vi "InitFromCfgFile.vi"(8 "error in (no error)":errorcluster, 10 "configuration file path":path) -> (0 "error out":errorcluster, 3 "ByteQXAPIBase out":refnum<class "ByteQXAPIBase.lvclass">)   [LabVIEW 2019, in "ByteQXWebAPI.lvlib" / "ByteQXAPIBase.lvclass"]
doc: "Initialize the api connection based on the path of an ini file containing the configuration\n[Server]\nAPI Root = \"\"\nVersion = \"\"\nPort = 0\nBase URL = \"\"\nVerify server =\nAuth type = \nTimeout = 10000\n\n[Token]\nAuth = \"\""
uses:
  ByteQXAPIBase.lvclass
  <vilib>/Utility/config.llb/Read Key (U32).vi
  <vilib>/Utility/config.llb/Read Key (String).vi
  <vilib>/Utility/config.llb/NI_LVConfig.lvlib
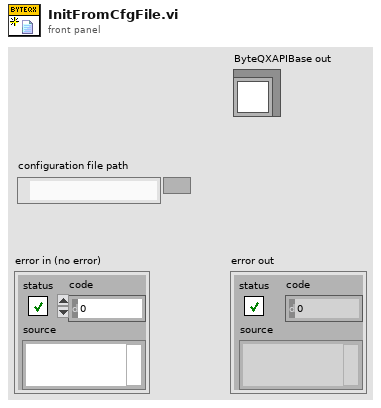
[diagram p1: front panel]
types:
  T1 = typedef "NI_LVConfig.lvlib/Config Data RefNum.ctl" = refnum<k1>
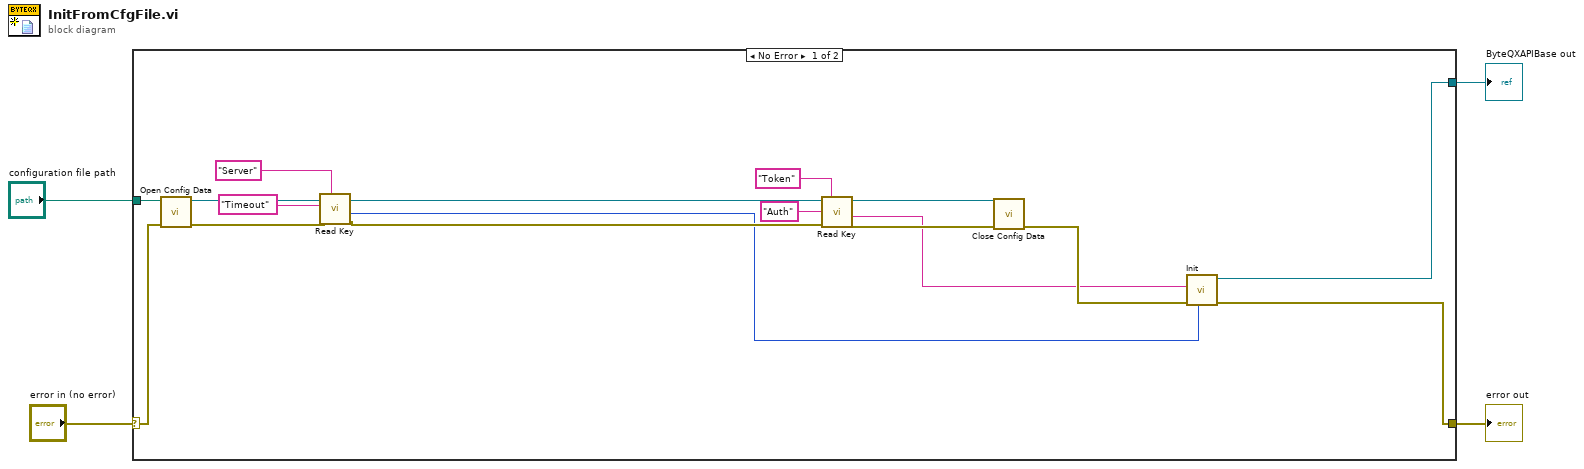
[diagram p0: block diagram]
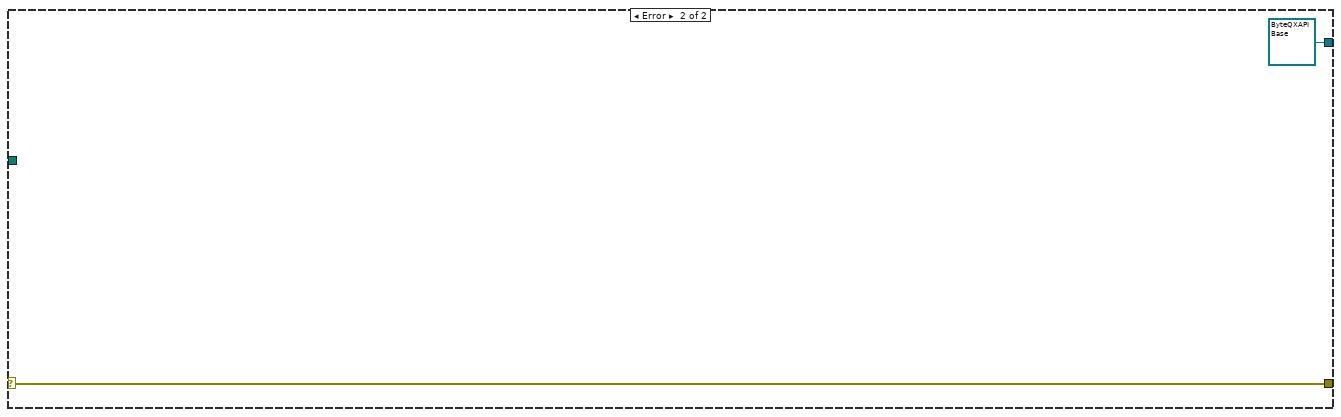
[diagram p2: hidden frame]
diagram:
  n1 = case shown="No Error" "error in (no error)" {
    selector: "error in (no error)" -> [w17 w23]
    tunnel: [w8 w23] -> w3
    tunnel: [w7 refnum<class "ByteQXAPIBase.lvclass"> refnum ("ByteQXAPIBase out")] -> w2
    tunnel: "configuration file path" -> [w19 _]
    frame No Error {
      n2 = call <vilib>:"Open Config Data.vi"("error in (no error)"=w17, "configuration file path"=w19) -> ("error out"=w21:errorcluster, "refnum"=w20:T1)  [unwired: 7 in, 1 out]
      n3 = call-poly <vilib>:"Read Key.vi"("section"="Server", "error in (no error)"=w21, "key"="Timeout", "refnum"=w20) -> ("error out"=w11:errorcluster, "value"=w6:u32, "refnum out"=w10:T1)  [unwired: 4 in, 1 out]
      n4 = call-poly <vilib>:"Read Key.vi"("section"="Token", "error in (no error)"=w11, "key"="Auth", "refnum"=w10) -> ("error out"=w13:errorcluster, "value"=w5:string, "refnum out"=w14:T1)  [unwired: 4 in, 1 out]
      n5 = call <vilib>:"Close Config Data.vi"("error in (no error)"=w13, "refnum"=w14) -> ("error out"=w9:errorcluster)  [unwired: 8 in, 1 out]
      n6 = call "Init.vi"("timeout (10000)"=w6, "error in (no error)"=w9, "Auth token"=w5) -> ("error out"=w8:errorcluster, "ByteQXAPIBase out"=w7:refnum<class "ByteQXAPIBase.lvclass">)  [unwired: 7 in]
    }
    frame Error {
    }
  }
  "error out" <- w3
  "ByteQXAPIBase out" <- w2
